vi "全局 所有参数.vi"() -> ()   [LabVIEW 2016, in "数据传输系统.lvlib"]
panel:
  in  "挥发酚加标回收率":string[][](array[string])
  in  "氯化物":string[][](array[string])
  in  "挥发酚":string[][](array[string])
  in  "氟化物加标回收率":string[][](array[string])
  in  "氟化物":string[][](array[string])
  in  "硝氮":string[][](array[string])
  in  "磷酸盐":string[][](array[string])
  in  "盐度 2":string[][](array[string])
  out "columns":string[](array[string])
  in  "风向":string[][](array[string])
  in  "风速":string[][](array[string])
  in  "气压":string[][](array[string])
  in  "气温":string[][](array[string])
  in  "汞":string[][](array[string])
  in  "锰":string[][](array[string])
  in  "镍":string[][](array[string])
  in  "锌":string[][](array[string])
  in  "ïÓ":string[][](array[string])
  in  "铅":string[][](array[string])
  in  "剖面多参数":string[][](array[string])
  in  "ORP":string[][](array[string])
  in  "硫化物":string[][](array[string])
  in  "亚硝酸盐":string[][](array[string])
  in  "总磷加标回收率":string[][](array[string])
  in  "总氮加标回收率":string[][](array[string])
  in  "氨氮加标回收率":string[][](array[string])
  in  "CODCr加标回收率":string[][](array[string])
  in  "CODMn加标回收率":string[][](array[string])
  in  "累积流量":string[][](array[string])
  in  "瞬时流量":string[][](array[string])
  in  "流速":string[][](array[string])
  in  "水位":string[][](array[string])
  in  "盐度":string[][](array[string])
  in  "铜":string[][](array[string])
  in  "藻密度":string[][](array[string])
  in  "叶绿素":string[][](array[string])
  in  "浊度":string[][](array[string])
  in  "DO":string[][](array[string])
  in  "水温":string[][](array[string])
  in  "电导率":string[][](array[string])
  in  "总磷":string[][](array[string])
  in  "总氮":string[][](array[string])
  in  "CODMn":string[][](array[string])
  in  "氨氮":string[][](array[string])
  in  "CODCr":string[][](array[string])
  in  "PH":string[][](array[string])
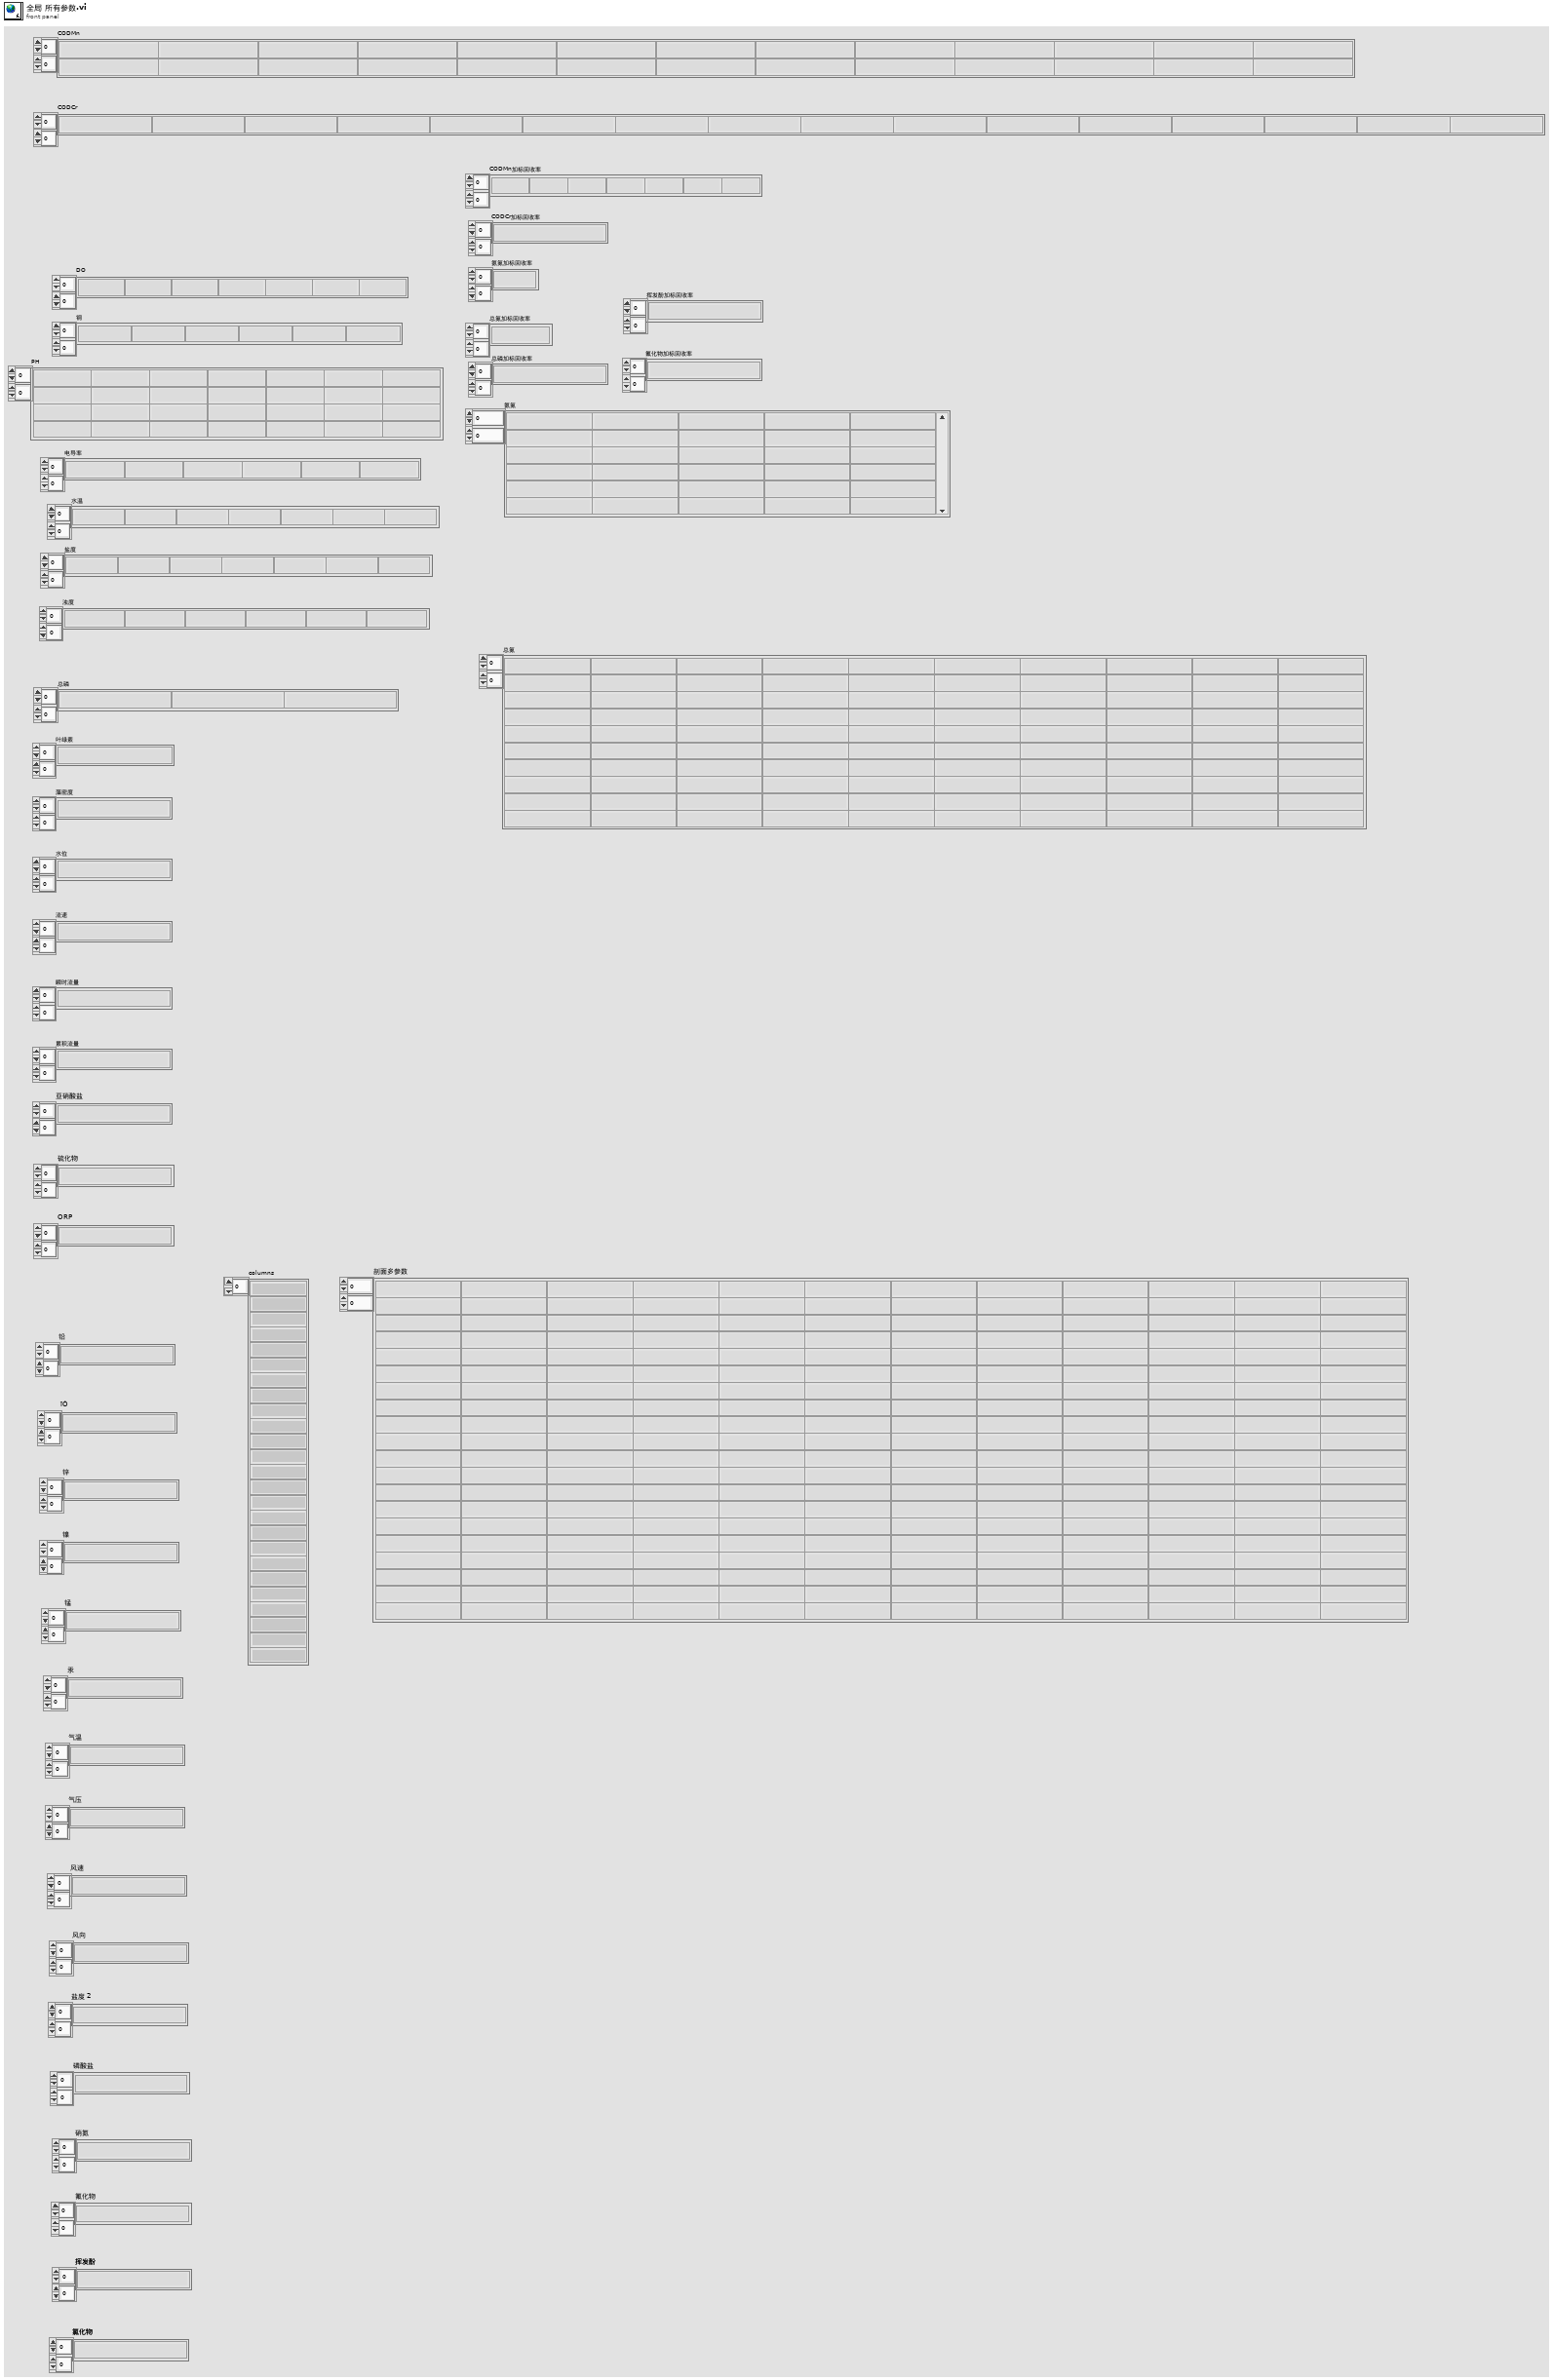
[diagram p1: front panel]
diagram:
